vi "Lesson5 - new type def.vi"() -> ()   [LabVIEW 2013]
uses:
  Lesson5 - new TypeDef.ctl
panel:
  in  "Cluster 2":T1
  in  "Cluster":T1
  # "1. right click on cluster > make Type Def\n2. right click again, > open Type Def > save as .ctl file\n3 .  >> can change to strict type def if want to change APPEARANCE (as well as datatype) of all instances by changing master copy (analogous to LaTeX commands vs hard-coding)"
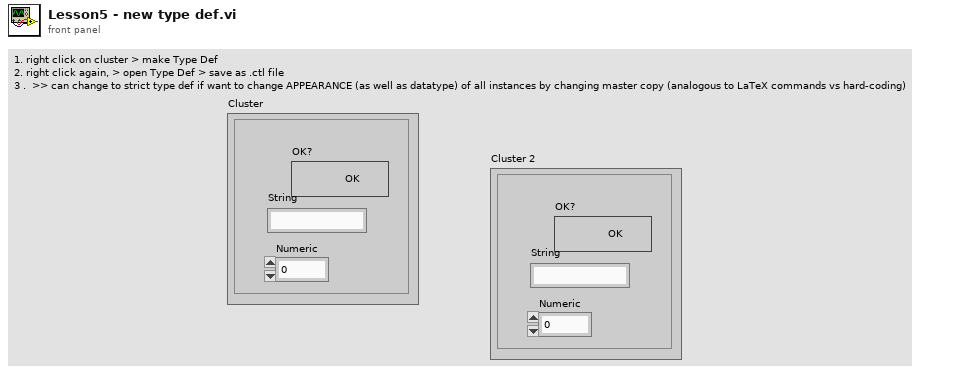
[diagram p1: front panel]
types:
  T1 = typedef "Lesson5 - new TypeDef.ctl" = cluster{"OK?":bool, "String":string, "Numeric":dbl}
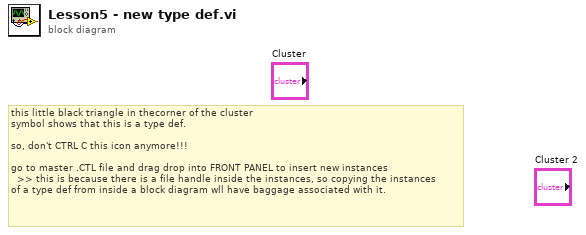
[diagram p0: block diagram]
diagram:
  # "this little black triangle in thecorner of the cluster \nsymbol shows that this is a type def.\n\nso, don't CTRL C this icon anymore!!!\n\ngo to master .CTL file and drag drop into FRONT PANEL to insert new instances\n  >> this is because there is a file handle inside the instances, so copying the instances\nof a type def from inside a block diagram wll have baggage associated with it."
